vi "Day12-1.vi"() -> ()   [LabVIEW 2021]
panel:
  out "finished paths":i32
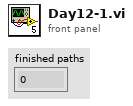
[diagram p1: front panel]
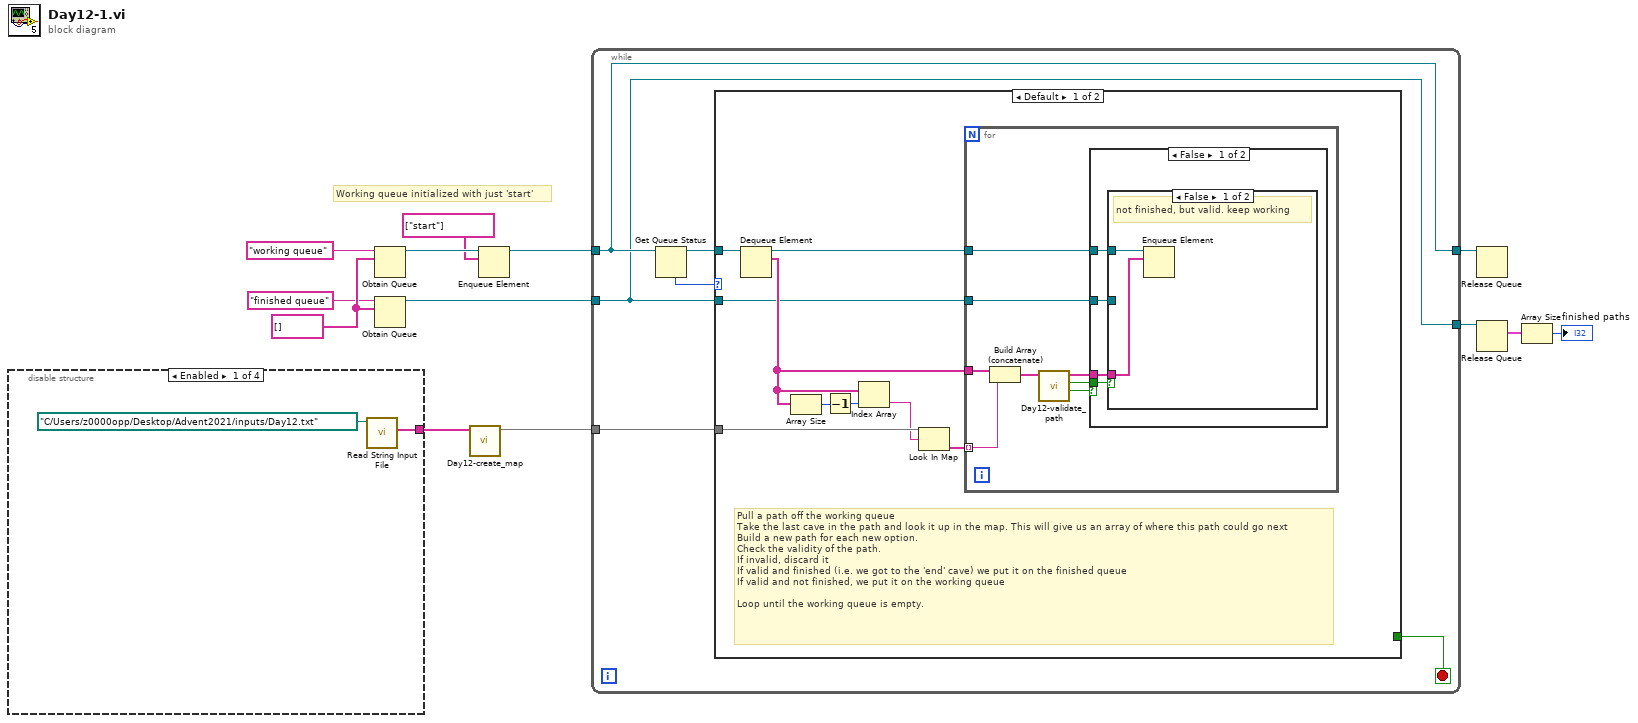
[diagram p0: block diagram]
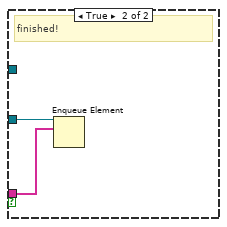
[diagram p2: hidden frame]
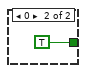
[diagram p4: hidden frame]
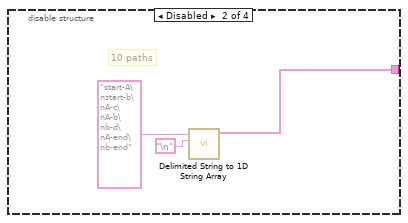
[diagram p5: hidden frame]
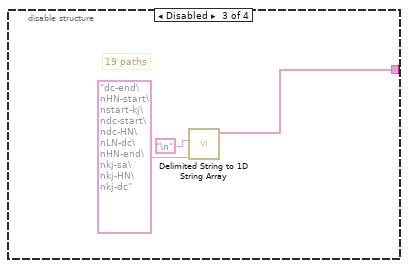
[diagram p6: hidden frame]
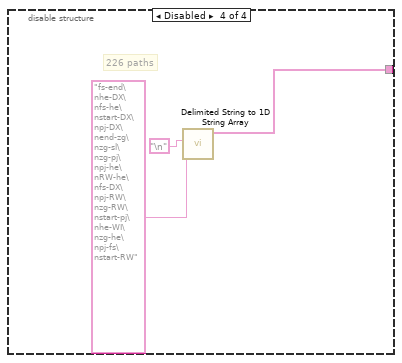
[diagram p7: hidden frame]
diagram:
  w10 = string[] []
  # "Working queue initialized with just 'start'"
  n1 = disable-structure shown="Enabled" {
    disable-tunnel: [w14 w16 w19 w22] -> w13
    frame Enabled {
      n2 = call "Read String Input File.vi"("file path (dialog if empty)"=path "C:/Users/z0000opp/Desktop/Advent2021/inputs/Day12.txt") -> ("input values"=w14:string[])  [unwired: 10 in]
    }
    frame Disabled {
      # "10 paths"
      n3 = call <vilib>:"Delimited String to 1D String Array.vi"("delimiter"="\n", "delimited string"="start-A\nstart-b\nA-c\nA-b\nb-d\nA-end\nb-end") -> ("string array"=w16:string[])  [unwired: 9 in]
    }
    frame Disabled {
      # "19 paths"
      n4 = call <vilib>:"Delimited String to 1D String Array.vi"("delimiter"="\n", "delimited string"="dc-end\nHN-start\nstart-kj\ndc-start\ndc-HN\nLN-dc\nHN-end\nkj-sa\nkj-HN\nkj-dc") -> ("string array"=w19:string[])  [unwired: 9 in]
    }
    frame Disabled {
      # "226 paths"
      n5 = call <vilib>:"Delimited String to 1D String Array.vi"("delimiter"="\n", "delimited string"="fs-end\nhe-DX\nfs-he\nstart-DX\npj-DX\nend-zg\nzg-sl\nzg-pj\npj-he\nRW-he\nfs-DX\npj-RW\nzg-RW\nstart-pj\nhe-WI\nzg-he\npj-fs\nstart-RW") -> ("string array"=w22:string[])  [unwired: 9 in]
    }
  }
  n6 = Obtain Queue(name (unnamed)="working queue", element data type=w10) -> (queue out=w12:refnum<queue>)  [unwired: 3 in, 2 out]
  n7 = Obtain Queue(name (unnamed)="finished queue", element data type=w10) -> (queue out=w5:refnum<queue>)  [unwired: 3 in, 2 out]
  n8 = call "Day12-create_map.vi"("string array"=w13) -> ("Map"=w7:map{string, string[]})  [unwired: 10 in]
  n9 = Enqueue Element(queue=w12, element=string[] ["start"]) -> (queue out=w6:refnum<queue>)  [unwired: 2 in, 2 out]
  n10 = while {
    tunnel: w7 -> [w27]
    tunnel: w6 -> [w26]
    tunnel: w5 -> [w25]
    tunnel: [w26] -> w4
    tunnel: [w25] -> w3
    stop <- w29 stop-if-true
    n11 = Get Queue Status(queue=w26) -> (queue out=w28:refnum<queue>, # elements in queue=w30:i32)  [unwired: 2 in, 6 out]
    n12 = case shown="Default" w30 {
      tunnel: [_ TRUE] -> w29
      tunnel: w28 -> [w39 _]
      tunnel: w25 -> [w31 _]
      tunnel: w27 -> [w36 _]
      frame Default {
        # "Pull a path off the working queue\nTake the last cave in the path and look it up in the map. This will give us an array of where this path could go next\nBuild a new path for each new option.\nCheck the validity of the path.\nIf invalid, discard it\nIf valid and finished (i.e. we got to the 'end' cave) we put it on the finished queue\nIf valid and not finished, we put it on the working queue\n\nLoop until the working queue is empty."
        n13 = Dequeue Element(queue=w39) -> (queue out=w32:refnum<queue>, element=w34:string[])  [unwired: 2 in, 2 out]
        n14 = Array Size(array=w34) -> (size(s)=w38:i32)
        n15 = Decrement(x=w38) -> (x-1=w37:i32)
        n16 = Index Array(array=w34, index=w37) -> (element=w35:string)
        n17 = Look In Map(map=w36, key=w35) -> (value=w33:string[])  [unwired: 1 in, 1 out]
        n18 = for {
          tunnel: w34 -> [w47]
          tunnel: w33 -> [w46] mode=indexing
          tunnel: w32 -> [w40]
          tunnel: w31 -> [w41]
          n19 = Build Array (concatenate)(w47, w46) -> (w45:string[])
          n20 = call "Day12-validate_path.vi"("Path"=w45) -> ("invalid?"=w44:bool, "finshed?"=w42:bool, "Path out"=w43:string[])  [unwired: 8 in]
          n21 = case shown="False" w44 {
            tunnel: w43 -> [w49 _]
            tunnel: w42 -> [w51 _]
            tunnel: w41 -> [w50 _]
            tunnel: w40 -> [w48 _]
            frame False {
              n22 = case shown="False" w51 {
                tunnel: w50 -> [_ w55]
                tunnel: w49 -> [w52 w54]
                tunnel: w48 -> [w53 _]
                frame False {
                  # "not finished, but valid. keep working"
                  n23 = Enqueue Element(queue=w53, element=w52) -> ()  [unwired: 2 in, 3 out]
                }
                frame True {
                  # "finished!"
                  n24 = Enqueue Element(queue=w55, element=w54) -> ()  [unwired: 2 in, 3 out]
                }
              }
            }
            frame True {
              # "invalid, do nothing"
            }
          }
        }
      }
      frame 0 {
      }
    }
  }
  n25 = Release Queue(queue=w4) -> ()  [unwired: 2 in, 3 out]
  n26 = Release Queue(queue=w3) -> (remaining elements=w2:cluster{string[]}[])  [unwired: 2 in, 2 out]
  n27 = Array Size(array=w2) -> (size(s)=→"finished paths":i32)
